vi "MainVI.vi"() -> ()   [LabVIEW 2013]
panel:
  out "Loop":i32
  in  "AsynchronousCall":bool
  in  "SubVI":bool
  # "我是MAIN VI"
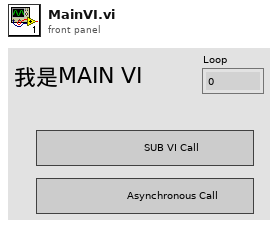
[diagram p1: front panel]
types:
  T1 = enum32{"Invalid", "Standard", "Closed", "Hidden", "Minimized", "Maximized"}
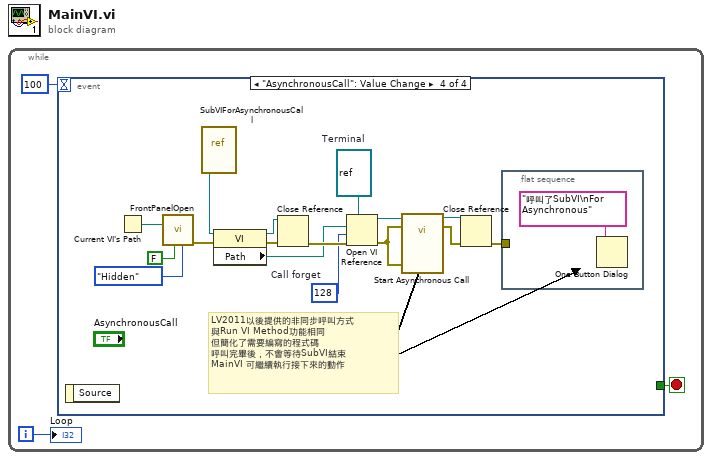
[diagram p0: block diagram]
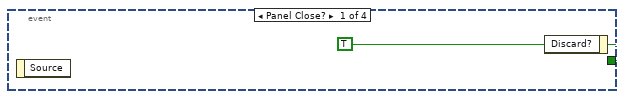
[diagram p2: hidden frame]
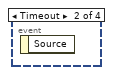
[diagram p3: hidden frame]
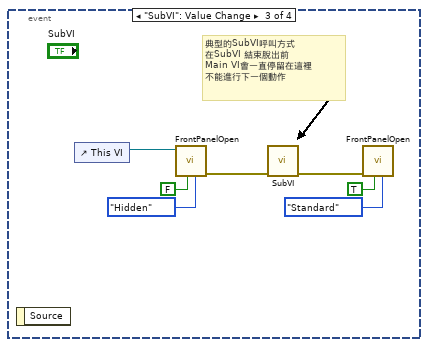
[diagram p4: hidden frame]
diagram:
  n1 = while {
    i -> [w2]
    stop <- w3 stop-if-true
    n2 = event shown="[3] \"AsynchronousCall\": Value Change" {
      selector: _ -> [_ _ _ _]
      dyn-events: _ -> [_ _ _ _]
      timeout: 100 -> [_ _ _ _]
      tunnel: [w4 _ _ _] -> w3
      event Panel Close? {
        w4 = TRUE ("Discard?")
        n3 = event-data() -> ()  [unwired: 1 in, 1 out]
        n4 = event-data("Discard?"=w4) -> ()  [unwired: 1 in, 1 out]
      }
      event Timeout {
        n5 = event-data() -> ()  [unwired: 1 in, 1 out]
      }
      event "SubVI": Value Change {
        # "典型的SubVI呼叫方式\n在SubVI 結束脫出前\nMain VI會一直停留在這裡\n不能進行下一個動作"
        n6 = event-data() -> ()  [unwired: 1 in, 1 out]
        n7 = control-ref of="This VI"() -> (w11:refnum<vi>)
        n8 = call "FrontPanelOpen.vi"("State"=T1."Hidden", "Activate?"=FALSE, "VI in"=w11) -> ("error out"=w8:errorcluster)  [unwired: 7 in, 1 out]
        n9 = call "SubVI.vi"("error in (no error)"=w8) -> ("error out"=w5:errorcluster)  [unwired: 10 in]
        n10 = call "FrontPanelOpen.vi"("State"=T1."Standard", "Activate?"=TRUE, "error in (no error)"=w5) -> ()  [unwired: 7 in, 2 out]
      }
      event "AsynchronousCall": Value Change {
        w13 = 128  # Call forget
        w18 = refnum<vi> refnum  # Terminal
        # "LV2011以後提供的非同步呼叫方式\n與Run VI Method功能相同\n但簡化了需要編寫的程式碼\n呼叫完畢後，不會等待SubVI結束\nMainVI 可繼續執行接下來的動作"
        n11 = event-data() -> ()  [unwired: 1 in, 1 out]
        n12 = Current VI's Path() -> (path=w25:path)
        n13 = call "FrontPanelOpen.vi"("State"=T1."Hidden", "Activate?"=FALSE, "VI Path"=w25) -> ("error out"=w21:errorcluster)  [unwired: 7 in, 1 out]
        n14 = vi-ref "SubVIForAsynchronousCall.vi"() -> (w24:refnum<vi>)
        n15 = property class="VI"(reference=w24, error in=w21) -> (reference out=w22:refnum<vi>, error out=w23:errorcluster, "Path"=w19:path)
        n16 = Close Reference(reference=w22, error in (no error)=w23) -> (error out=w20:errorcluster)
        n17 = Open VI Reference(type specifier VI Refnum (for type only)=w18, vi path=w19, options=w13, error in (no error)=w20) -> (vi reference=w17:refnum<vi>, error out=w16:errorcluster)  [unwired: 2 in]
        n18 = call-by-ref "Start Asynchronous Call"(reference=w17, error in=w16, 8:"error in (no error)"=w16) -> (reference out=w14:refnum<vi>, error out=w15:errorcluster)  [unwired: 10 in, 1 out]
        n19 = Close Reference(reference=w14, error in (no error)=w15) -> (error out=w12:errorcluster)
        n20 = flat-sequence {
          tunnel: w12 -> [_]
          frame #0 {
            n21 = One Button Dialog(message="呼叫了SubVI\nFor Asynchronous") -> ()  [unwired: 1 in, 1 out]
          }
        }
      }
    }
    "Loop" <- w2
  }
